vi "Volt_to_Angle.vi"(0 "Voltaje IN":dbl min=0.0 max=5.0 step=0.01, 11 "Error In":errorcluster) -> (4 "Angulo OUT":dbl, 15 "Error Out":errorcluster)   [LabVIEW 2016]
panel:
  in  "OK":bool
  out "Voltaje OUT":dbl
  in  "Angulo IN":dbl
  # "Conversión Voltaje -> Ángulo"
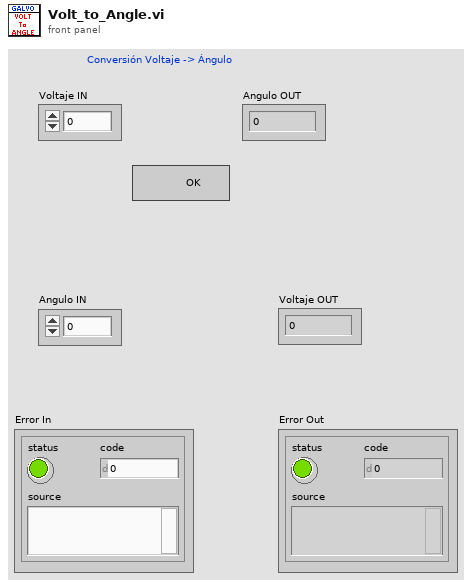
[diagram p1: front panel]
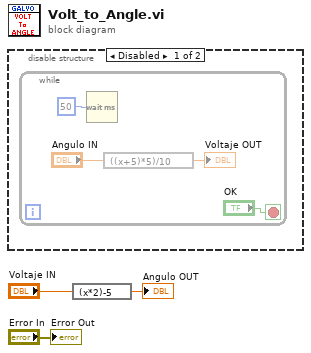
[diagram p0: block diagram]
diagram:
  n1 = disable-structure shown="Disabled" {
    frame Disabled {
      n2 = while {
        stop <- "OK" stop-if-true
        n3 = Wait (ms)(milliseconds to wait=u32 50) -> ()  [unwired: 1 out]
        n4 = expression code="((x+5)*5)/10"("Angulo IN") -> (→"Voltaje OUT":dbl)
      }
    }
    frame Enabled {
    }
  }
  n5 = expression code="(x*2)-5"("Voltaje IN") -> (→"Angulo OUT":dbl)
  "Error Out" <- "Error In"
